vi "Create Instance Impl.vi"(8 "error in (no error)":errorcluster, 10 "Fluidics Configuration":T1={"Serial Port"="COM3", "Device Type"=enum."Disabled"}, 11 "Autosampler in":refnum<class "Autosampler.lvclass">) -> (0 "error out":errorcluster, 3 "Autosampler out":refnum<class "Autosampler.lvclass">)   [LabVIEW 2023, in "Autosampler.lvlib" / "Autosampler.lvclass"]
uses:
  Autosampler.lvclass
  Resources/Type Defs/Autosampler Configuration.ctl
  Autosampler.lvclass/Autosampler.ctl
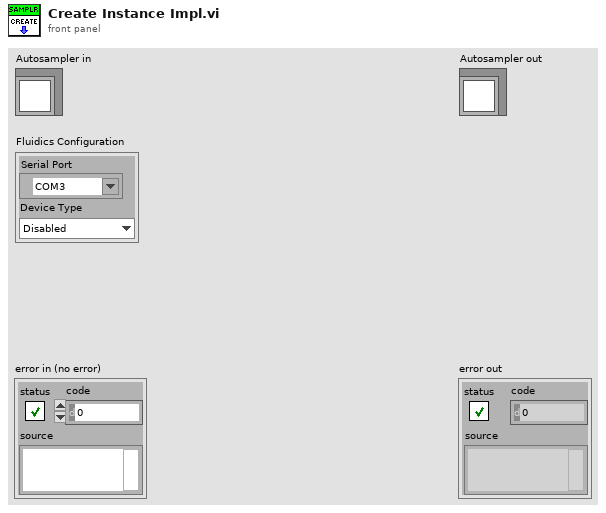
[diagram p1: front panel]
types:
  T1 = typedef "Autosampler Configuration.ctl" = cluster{"Serial Port":refnum<visa-resource-name>, "Device Type":enum16{"Disabled", "Simulate", "Alltesta"}}
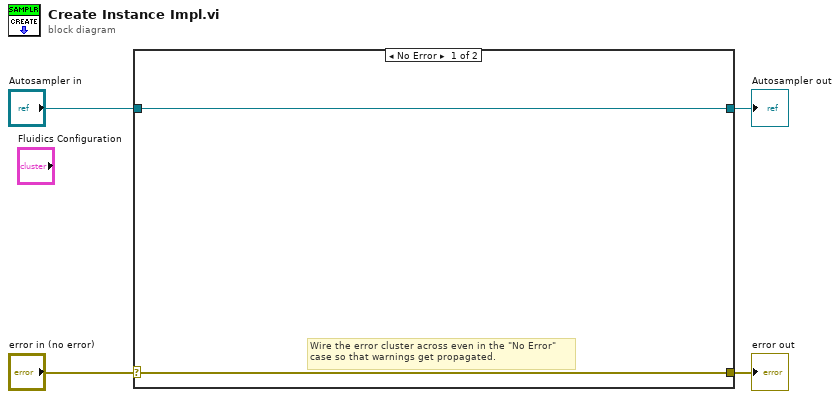
[diagram p0: block diagram]
diagram:
  n1 = case shown="No Error" "error in (no error)" {
    selector: "error in (no error)" -> [w5 w8]
    tunnel: [w5 w8] -> w3
    tunnel: [w6 w7] -> w1
    tunnel: "Autosampler in" -> [w6 w7]
    frame No Error {
      # "Wire the error cluster across even in the \"No Error\"\ncase so that warnings get propagated."
    }
    frame Error {
    }
  }
  "error out" <- w3
  "Autosampler out" <- w1
